vi "Configure Test Settings.vi"(8 "error in (no error)":errorcluster, 10 "Test Settings":T2={"Resistivity"=enum."Low", "Compliance Level (Volts)"=0.0, "Current Level (Amps)"=0.0, "Soak Time (Seconds)"=0.0, "Sample Thickness (cm)"=0.0, "Magnetic Flux (Gauss)"=0.0, "NPLC Ammeter"=1.0, "Count Ammeter"=1, "NPLC Voltmeter"=1.0, "Count Voltmeter"=1, "Sample Dimensions x"=0.0, "Sample Dimensions y"=0.0, "Sample Dimensions D1"=0.0, "Sample Dimensions D2"=0.0, "Sample Width Ws"=0.0, "Slot Number of 3765 Card"=0} {"Count Voltmeter" min=1 max=1024; "NPLC Voltmeter" min=0.001 max=10.0; "Count Ammeter" min=1 max=1024; "NPLC Ammeter" min=0.001 max=10.0}) -> (0 "error out":errorcluster)   [LabVIEW 2016, in "Hall Effect Library.lvlib"]
uses:
  Hall Effect Library.lvlib
  Controls/Resisitivity.ctl
  Private/Global Variables/Test Settings.vi
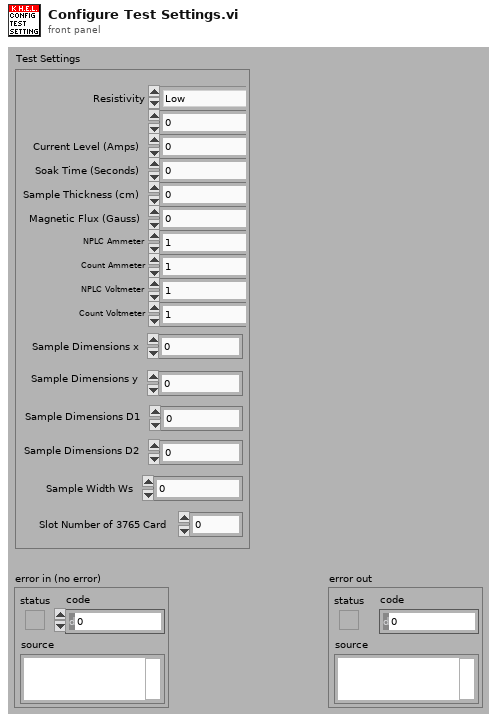
[diagram p1: front panel]
types:
  T1 = typedef "Hall Effect Library.lvlib/Resisitivity.ctl" = enum16{"Low", "High"}
  T2 = cluster{"Resistivity":T1, "Compliance Level (Volts)":dbl, "Current Level (Amps)":dbl, "Soak Time (Seconds)":dbl, "Sample Thickness (cm)":dbl, "Magnetic Flux (Gauss)":dbl, "NPLC Ammeter":dbl, "Count Ammeter":i32, "NPLC Voltmeter":dbl, "Count Voltmeter":i32, "Sample Dimensions x":dbl, "Sample Dimensions y":dbl, "Sample Dimensions D1":dbl, "Sample Dimensions D2":dbl, "Sample Width Ws":dbl, "Slot Number of 3765 Card":u8}
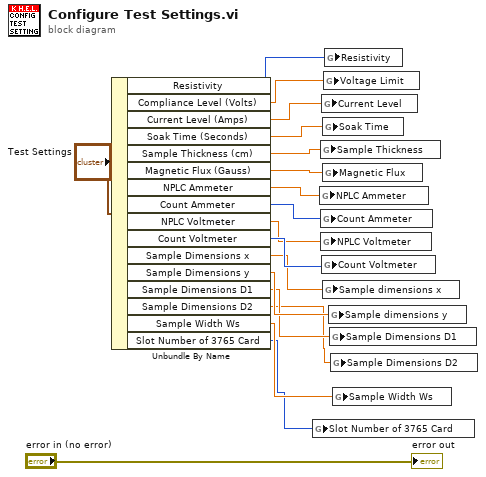
[diagram p0: block diagram]
diagram:
  n1 = Unbundle By Name("Test Settings") -> ("Resistivity"=w14:T1, "Compliance Level (Volts)"=w9:dbl, "Current Level (Amps)"=w8:dbl, "Soak Time (Seconds)"=w7:dbl, "Sample Thickness (cm)"=w15:dbl, "Magnetic Flux (Gauss)"=w16:dbl, "NPLC Ammeter"=w10:dbl, "Count Ammeter"=w11:i32, "NPLC Voltmeter"=w12:dbl, "Count Voltmeter"=w13:i32, "Sample Dimensions x"=w6:dbl, "Sample Dimensions y"=w5:dbl, "Sample Dimensions D1"=w4:dbl, "Sample Dimensions D2"=w3:dbl, "Sample Width Ws"=w2:dbl, "Slot Number of 3765 Card"=w1:u8)
  n2 = global write "Test Settings.vi" "Slot Number of 3765 Card"(w1) -> ()
  n3 = global write "Test Settings.vi" "NPLC Ammeter"(w10) -> ()
  n4 = global write "Test Settings.vi" "Sample Thickness"(w15) -> ()
  n5 = global write "Test Settings.vi" "Count Ammeter"(w11) -> ()
  n6 = global write "Test Settings.vi" "NPLC Voltmeter"(w12) -> ()
  n7 = global write "Test Settings.vi" "Current Level"(w8) -> ()
  n8 = global write "Test Settings.vi" "Count Voltmeter"(w13) -> ()
  n9 = global write "Test Settings.vi" "Soak Time"(w7) -> ()
  n10 = global write "Test Settings.vi" "Magnetic Flux"(w16) -> ()
  n11 = global write "Test Settings.vi" "Sample dimensions x"(w6) -> ()
  n12 = global write "Test Settings.vi" "Voltage Limit"(w9) -> ()
  n13 = global write "Test Settings.vi" "Resistivity"(w14) -> ()
  n14 = global write "Test Settings.vi" "Sample dimensions y"(w5) -> ()
  n15 = global write "Test Settings.vi" "Sample Dimensions D1"(w4) -> ()
  n16 = global write "Test Settings.vi" "Sample Dimensions D2"(w3) -> ()
  n17 = global write "Test Settings.vi" "Sample Width Ws"(w2) -> ()
  "error out" <- "error in (no error)"
